vi "multiVi_test.vi"() -> ()   [LabVIEW 2016]
uses:
  global/Config_Infos.vi
panel:
  in  "x":bool
  in  "Tab Control":T1(tab)
  out "Init OK?":bool
  out "error initialization (out)":errorcluster
  out "broadcast.ping listener?":bool
  out "broadcast.ping listener? 2":bool
  out "broadcast.ping error out":errorcluster
  out "Execution:State":T2(ring)
  out "ping error out":errorcluster
  out "broadcast.ping error out 2":errorcluster
  out "ping error out 2":errorcluster
  out "Execution:State 2":T2(ring)
  in  "config file":path=path "C:/Users/project8/Documents/SourceTree/hardware/software_config/rga/RGAConfig.ini"
  in  "stop":bool
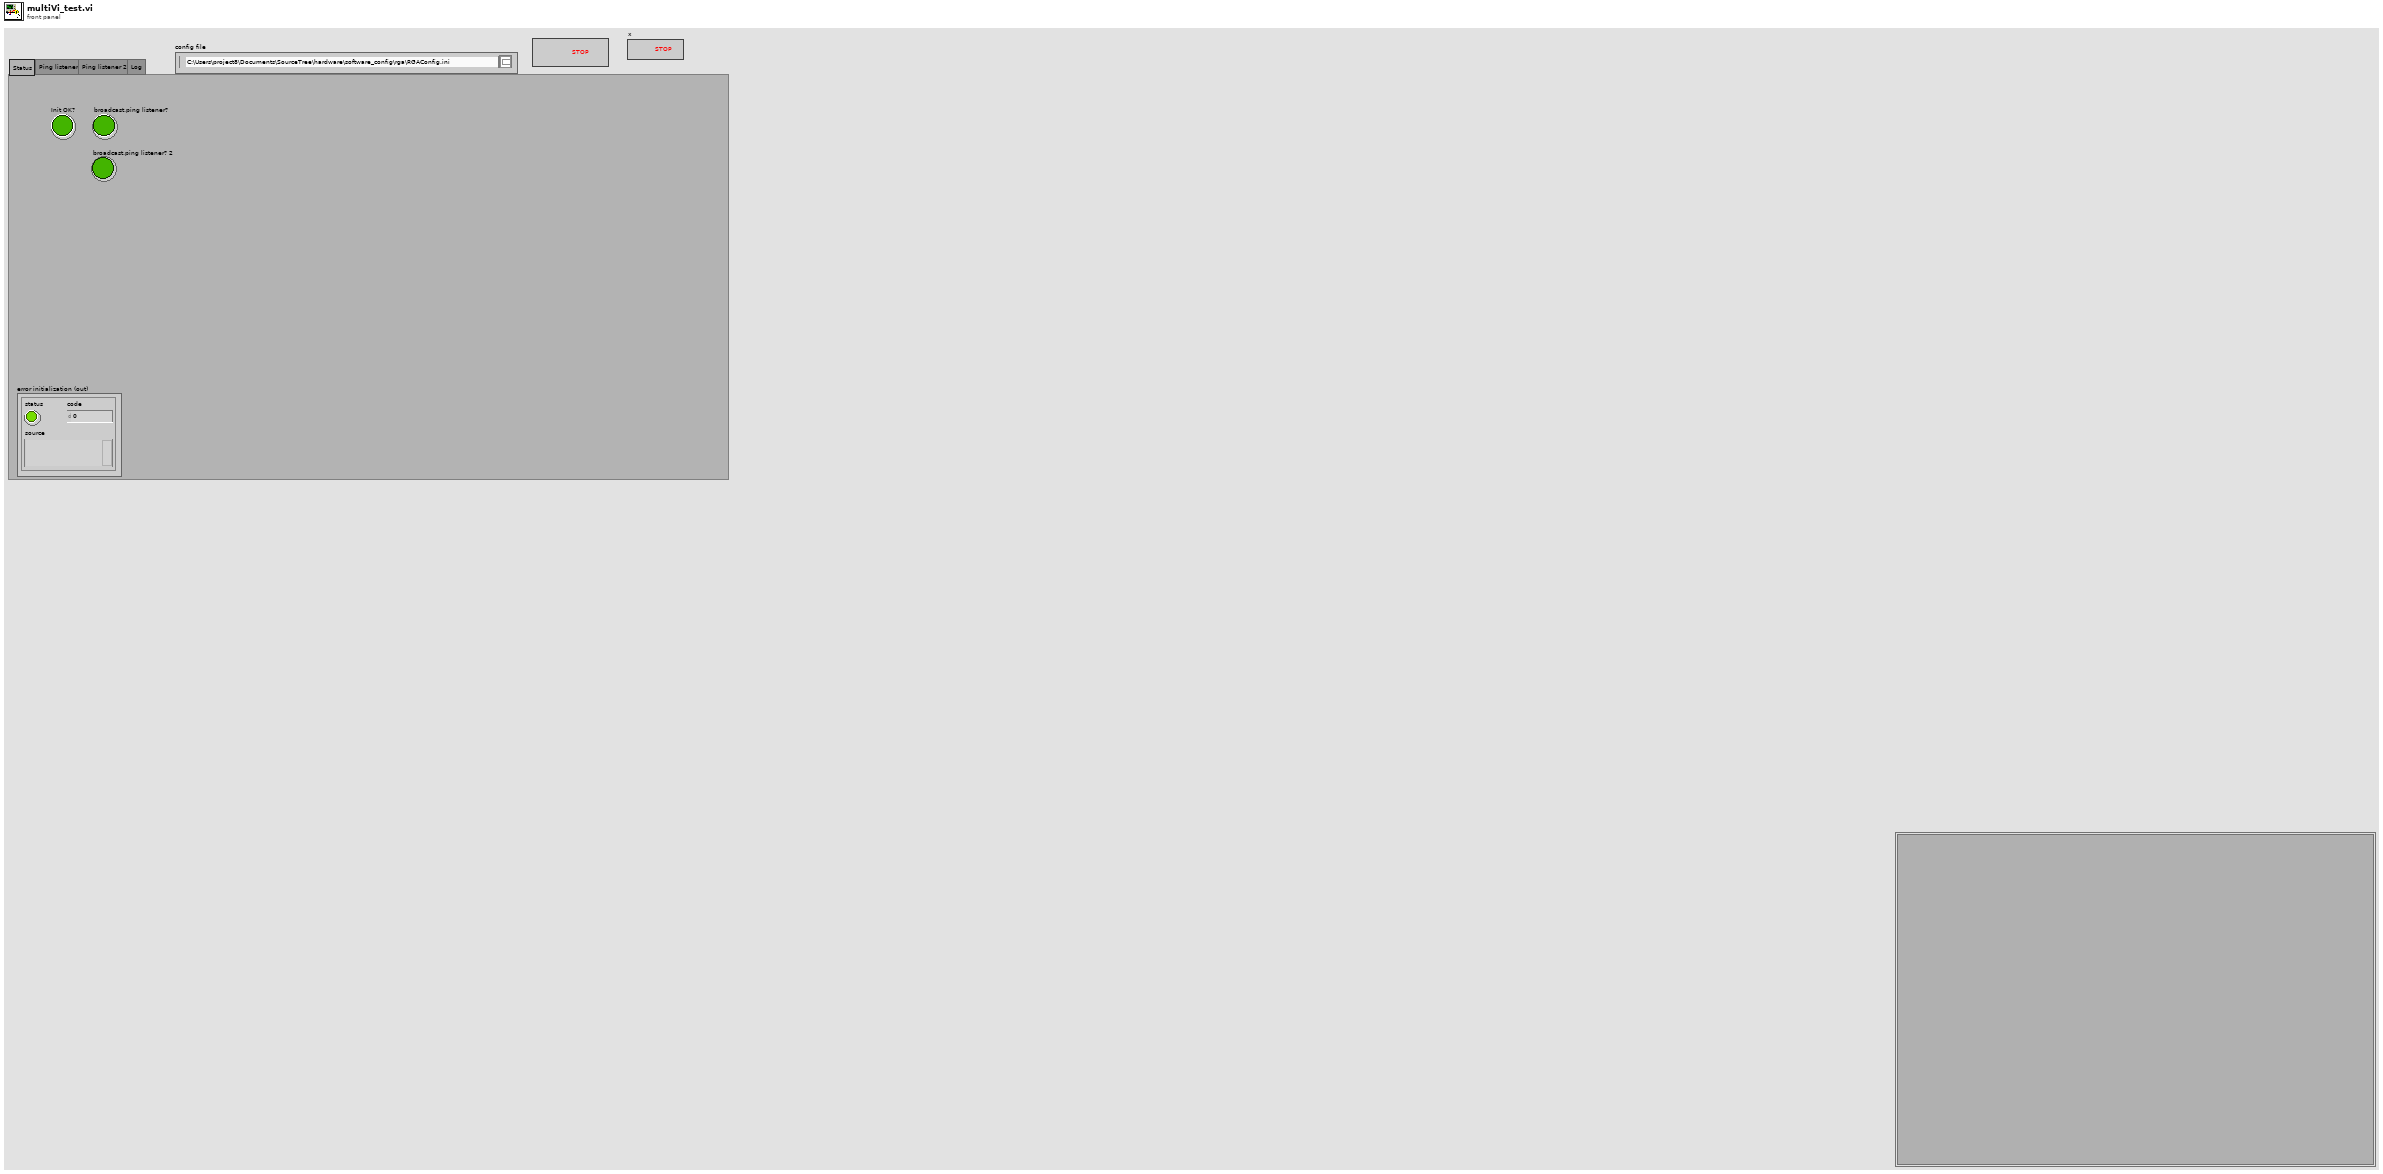
[diagram p1: front panel]
types:
  T1 = enum32{"Status", "Ping listener", "Ping listener 2", "Log"}
  T2 = enum32{"Bad", "Idle", "Run top level", "Running"}
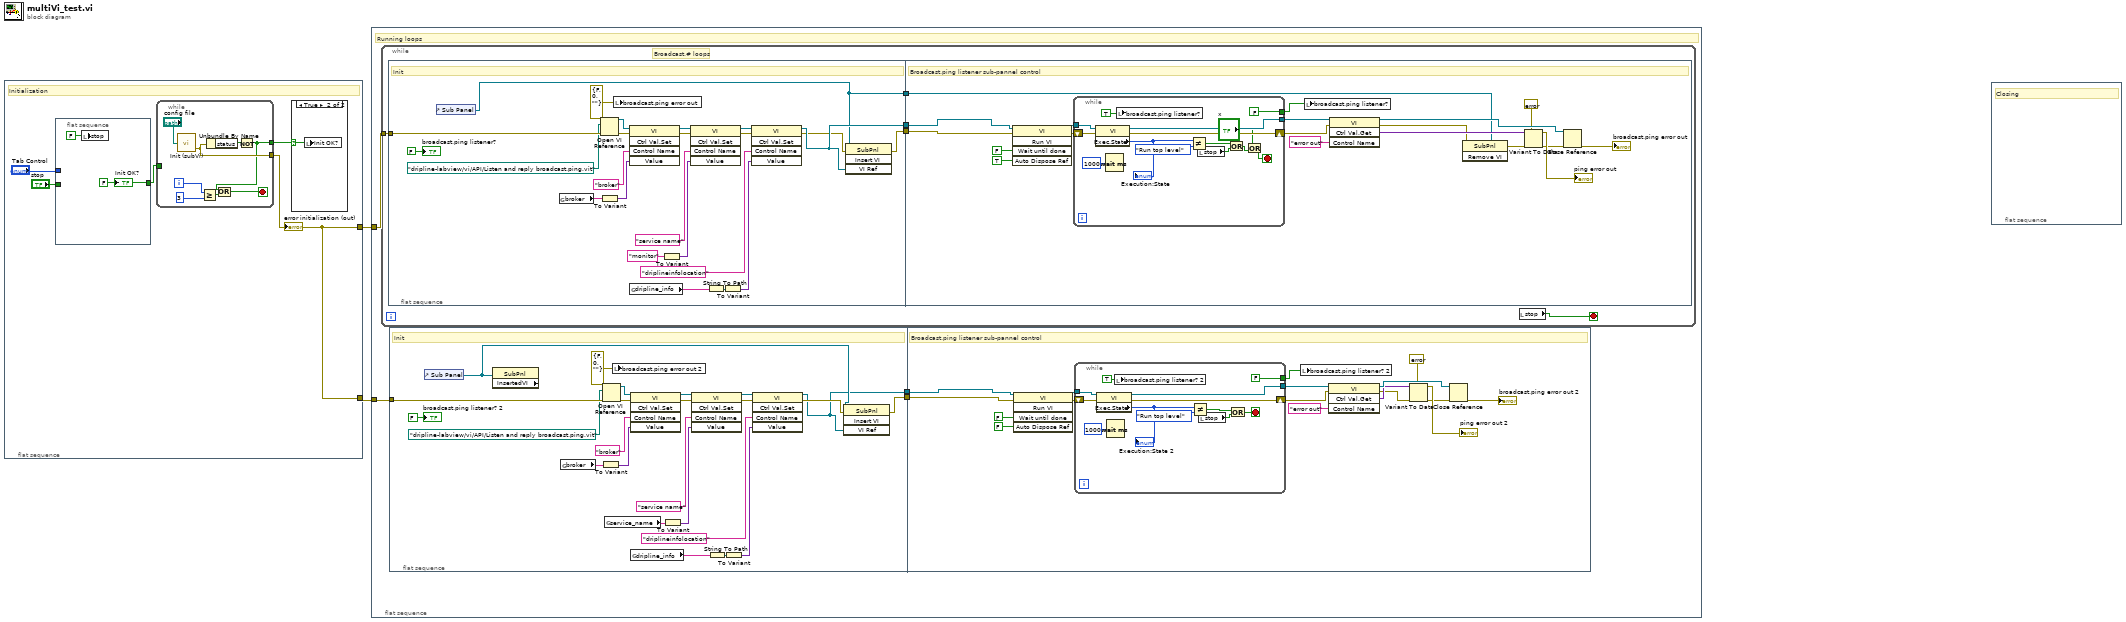
[diagram p0: block diagram]
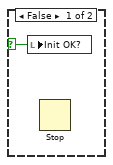
[diagram p2: hidden frame]
diagram:
  n1 = flat-sequence {
    tunnel: [w3] -> w2
    tunnel: [w3] -> w1
    frame #0 {
      # "Initialization"
      n2 = flat-sequence {
        tunnel: [w9] -> w6
        tunnel: "stop" -> [_]
        tunnel: "Tab Control" -> [_]
        frame #0 {
          w9 = FALSE ("Init OK?")
          n3 = local write "stop"(FALSE ("stop")) -> ()
          "Init OK?" <- w9
        }
      }
      n4 = while {
        tunnel: [w13] -> w7
        tunnel: [w14] -> w3
        tunnel: w6 -> [_]
        i -> [w17]
        stop <- w19 stop-if-true
        n5 = call "Init (subVi).vi"("config file"="config file") -> ("error (out)"=w14:errorcluster)  [unwired: 2 in]
        n6 = Greater Or Equal?(x=w17, y=3) -> (x >= y?=w18:bool)
        n7 = Unbundle By Name(w14) -> ("status"=w15:bool)
        n8 = Not(x=w15) -> (.not. x?=w13:bool)
        n9 = Or(x=w13, y=w18) -> (x .or. y?=w19:bool)
      }
      "error initialization (out)" <- w3
      n10 = case shown="True" w7 {
        selector: w7 -> [w10 w11]
        frame False {
          n11 = local write "Init OK?"(w10) -> ()
          n12 = Stop() -> ()  [unwired: 1 in]
        }
        frame True {
          n13 = local write "Init OK?"(w11) -> ()
        }
      }
    }
  }
  n14 = flat-sequence {
    tunnel: w2 -> [w23]
    tunnel: w1 -> [w20]
    frame #0 {
      # "Running loops"
      n15 = while {
        tunnel: w23 -> [w26]
        stop <- w25 stop-if-true
        # "Broadcast.# loops"
        n16 = flat-sequence {
          tunnel: w26 -> [w47]
          tunnel: [w32] -> w28
          tunnel: [w30] -> w27
          tunnel: [w29] -> w24
          tunnel: w28 -> [w59]
          tunnel: w27 -> [w60]
          tunnel: w24 -> [w53]
          frame #0 {
            # "Init"
            n17 = control-ref of="Sub Panel"() -> (w29:refnum<vi>)
            n18 = global read "Config_Infos.vi" "broker"() -> (w49:string)
            n19 = Open VI Reference(vi path=path "dripline-labview/vi/API/Listen and reply broadcast.ping.vit", error in (no error)=w47) -> (vi reference=w43:refnum<vi>, error out=w50:errorcluster)  [unwired: 4 in]
            n20 = To Variant(anything=w49) -> (Variant=w51:variant)
            n21 = local write "broadcast.ping error out"(errorcluster {"status"=FALSE, "code"=0, "source"=""} ("broadcast.ping error out")) -> ()
            n22 = invoke class="VI" method="Ctrl Val.Set"(reference=w43, error in=w50, "Control Name"="broker", "Value"=w51) -> (reference out=w45:refnum<vi>, error out=w44:errorcluster)  [unwired: 1 in, 3 out]
            n23 = global read "Config_Infos.vi" "dripline_info"() -> (w40:string)
            n24 = To Variant(anything="monitor") -> (Variant=w38:variant)
            n25 = invoke class="VI" method="Ctrl Val.Set"(reference=w45, error in=w44, "Control Name"="service name", "Value"=w38) -> (reference out=w34:refnum<vi>, error out=w42:errorcluster)  [unwired: 1 in, 3 out]
            n26 = String To Path(string=w40) -> (path=w35:path)
            n27 = To Variant(anything=w35) -> (Variant=w39:variant)
            n28 = invoke class="VI" method="Ctrl Val.Set"(reference=w34, error in=w42, "Control Name"="driplineinfolocation", "Value"=w39) -> (reference out=w32:refnum<vi>, error out=w31:errorcluster)  [unwired: 1 in, 3 out]
            n29 = invoke class="SubPnl" method="Insert VI"(reference=w29, error in=w31, "VI Ref"=w32) -> (error out=w30:errorcluster)  [unwired: 1 in, 3 out]
            "broadcast.ping listener?" <- FALSE ("Boolean")
          }
          frame #1 {
            # "Broadcast.ping listener sub-pannel control"
            n30 = invoke class="VI" method="Run VI"(reference=w59, error in=w60, "Wait until done"=FALSE ("Wait Until Done"), "Auto Dispose Ref"=TRUE ("Auto Dispose Reference")) -> (reference out=w57:refnum<vi>, error out=w55:errorcluster)  [unwired: 1 in, 3 out]
            n31 = while {
              tunnel: w57 -> [w83]
              tunnel: [w82] -> w71
              tunnel: [FALSE] -> w69
              shift-right: [w75] -> w63
              shift-left: w55 -> [w76]
              stop <- w73 stop-if-true
              n32 = property class="VI"(reference=w83, error in=w76) -> (reference out=w82:refnum<vi>, error out=w75:errorcluster, "Exec.State"=w80:T2)
              "Execution:State" <- w80
              n33 = Wait (ms)(milliseconds to wait=u32 1000) -> ()  [unwired: 1 out]
              n34 = local write "broadcast.ping listener?"(TRUE ("broadcast.ping listener?")) -> ()
              n35 = Not Equal?(x=w80, y=T2."Run top level") -> (x != y?=w77:bool)
              n36 = local read "stop"() -> (w81:bool)
              n37 = Or(x=w77, y=w81) -> (x .or. y?=w78:bool)
              n38 = Or(x="x", y=w78) -> (x .or. y?=w73:bool)
            }
            n39 = local write "broadcast.ping listener?"(w69) -> ()
            n40 = invoke class="VI" method="Ctrl Val.Get"(reference=w71, error in=w63, "Control Name"="error out") -> (reference out=w68:refnum<vi>, error out=w62:errorcluster, "Get Control Value Variant"=w66:variant)  [unwired: 1 in, 1 out]
            n41 = invoke class="SubPnl" method="Remove VI"(reference=w53, error in=w62) -> (error out=w54:errorcluster)  [unwired: 1 in, 2 out]
            n42 = Variant To Data(error in=w54, type=errorcluster {"status"=FALSE, "code"=0, "source"=""} ("broadcast.ping error out"), Variant=w66) -> (data=→"ping error out":errorcluster, error out=w61:errorcluster)
            n43 = Close Reference(reference=w68, error in (no error)=w61) -> (error out=→"broadcast.ping error out":errorcluster)
          }
        }
        n44 = local read "stop"() -> (w25:bool)
      }
      n45 = flat-sequence {
        tunnel: w20 -> [w109]
        tunnel: [w87] -> w22
        tunnel: [w86] -> w21
        tunnel: w22 -> [w125]
        tunnel: w21 -> [w126]
        frame #0 {
          # "Init"
          n46 = control-ref of="Sub Panel"() -> (w89:refnum<vi>)
          n47 = property class="SubPnl" props=["InsertedVI"](reference=w89) -> ()  [unwired: 1 in, 3 out]
          n48 = global read "Config_Infos.vi" "broker"() -> (w105:string)
          n49 = Open VI Reference(vi path=path "dripline-labview/vi/API/Listen and reply broadcast.ping.vit", error in (no error)=w109) -> (vi reference=w100:refnum<vi>, error out=w106:errorcluster)  [unwired: 4 in]
          n50 = To Variant(anything=w105) -> (Variant=w107:variant)
          n51 = global read "Config_Infos.vi" "service_name"() -> (w98:string)
          n52 = local write "broadcast.ping error out 2"(errorcluster {"status"=FALSE, "code"=0, "source"=""} ("broadcast.ping error out")) -> ()
          n53 = invoke class="VI" method="Ctrl Val.Set"(reference=w100, error in=w106, "Control Name"="broker", "Value"=w107) -> (reference out=w102:refnum<vi>, error out=w101:errorcluster)  [unwired: 1 in, 3 out]
          n54 = global read "Config_Infos.vi" "dripline_info"() -> (w97:string)
          n55 = To Variant(anything=w98) -> (Variant=w95:variant)
          n56 = invoke class="VI" method="Ctrl Val.Set"(reference=w102, error in=w101, "Control Name"="service name", "Value"=w95) -> (reference out=w91:refnum<vi>, error out=w99:errorcluster)  [unwired: 1 in, 3 out]
          n57 = String To Path(string=w97) -> (path=w92:path)
          n58 = To Variant(anything=w92) -> (Variant=w96:variant)
          n59 = invoke class="VI" method="Ctrl Val.Set"(reference=w91, error in=w99, "Control Name"="driplineinfolocation", "Value"=w96) -> (reference out=w87:refnum<vi>, error out=w88:errorcluster)  [unwired: 1 in, 3 out]
          n60 = invoke class="SubPnl" method="Insert VI"(reference=w89, error in=w88, "VI Ref"=w87) -> (error out=w86:errorcluster)  [unwired: 1 in, 3 out]
          "broadcast.ping listener? 2" <- FALSE ("Boolean")
        }
        frame #1 {
          # "Broadcast.ping listener sub-pannel control"
          n61 = invoke class="VI" method="Run VI"(reference=w125, error in=w126, "Wait until done"=FALSE ("Wait Until Done"), "Auto Dispose Ref"=FALSE ("Auto Dispose Reference")) -> (reference out=w123:refnum<vi>, error out=w118:errorcluster)  [unwired: 1 in, 3 out]
          n62 = while {
            tunnel: w123 -> [w136]
            tunnel: [w135] -> w122
            tunnel: [FALSE] -> w119
            shift-right: [w128] -> w112
            shift-left: w118 -> [w129]
            stop <- w131 stop-if-true
            n63 = property class="VI"(reference=w136, error in=w129) -> (reference out=w135:refnum<vi>, error out=w128:errorcluster, "Exec.State"=w133:T2)
            "Execution:State 2" <- w133
            n64 = Wait (ms)(milliseconds to wait=u32 1000) -> ()  [unwired: 1 out]
            n65 = local write "broadcast.ping listener? 2"(TRUE ("broadcast.ping listener?")) -> ()
            n66 = Not Equal?(x=w133, y=T2."Run top level") -> (x != y?=w130:bool)
            n67 = local read "stop"() -> (w134:bool)
            n68 = Or(x=w130, y=w134) -> (x .or. y?=w131:bool)
          }
          n69 = local write "broadcast.ping listener? 2"(w119) -> ()
          n70 = invoke class="VI" method="Ctrl Val.Get"(reference=w122, error in=w112, "Control Name"="error out") -> (reference out=w117:refnum<vi>, error out=w111:errorcluster, "Get Control Value Variant"=w115:variant)  [unwired: 1 in, 1 out]
          n71 = Variant To Data(error in=w111, type=errorcluster {"status"=FALSE, "code"=0, "source"=""} ("broadcast.ping error out"), Variant=w115) -> (data=→"ping error out 2":errorcluster, error out=w110:errorcluster)
          n72 = Close Reference(reference=w117, error in (no error)=w110) -> (error out=→"broadcast.ping error out 2":errorcluster)
        }
      }
    }
  }
  n73 = flat-sequence {
    frame #0 {
      # "Closing"
    }
  }
